vi "Out_Off_N4_201.vi"(4 "Driver Name":T10, 6 "Error Code":T11, 7 "SwitchOFF":T7=TRUE, 8 "error in":T9, 11 "DriverConnect in":T1={"InterfaceType"=enum."VISA", "OpenedSession"="", "InterfaceSettings"={"Interface"=enum."RS232", "EOS 4 read"=enum."LF (\\n)", "EOS 4 write"=enum."LF (\\n)", "TMO, ms"=10000, "Sett"=variant(cluster{"Baud Rate":u32, "Data Bits":u16, "Parity":u16, "Stop Bits":u16, "Flow Control":u16, "Eho":bool} {"Baud Rate"=75, "Data Bits"=0, "Parity"=0, "Stop Bits"=0, "Flow Control"=0, "Eho"=FALSE})}}) -> (0 "error out":T9, 3 "DriverConnect out":T1={"InterfaceType"=enum."VISA", "OpenedSession"="", "InterfaceSettings"={"Interface"=enum."RS232", "EOS 4 read"=enum."LF (\\n)", "EOS 4 write"=enum."LF (\\n)", "TMO, ms"=10000, "Sett"=variant(cluster{"Baud Rate":u32, "Data Bits":u16, "Parity":u16, "Stop Bits":u16, "Flow Control":u16, "Eho":bool} {"Baud Rate"=75, "Data Bits"=0, "Parity"=0, "Stop Bits"=0, "Flow Control"=0, "Eho"=FALSE})}})   [LabVIEW 2018]
uses:
  MOKO_LabViewLibrary/MokoLowLevel/MokoLowLovelControl/MLLC_ErrorCode.ctl
  MOKO_LabViewLibrary/MokoLowLevel/MokoLowLovelControl/MLLC_DriverName.ctl
  MOKO_LabViewLibrary/MokoLowLevel/MokoLowLovelControl/MLLC_Error.ctl
  MOKO_LabViewLibrary/MokoLowLevel/MokoLowLovelControl/MLLC_Delay.ctl
  MOKO_LabViewLibrary/MokoLowLevel/MokoLowLovelControl/MLLC_Boolean.ctl
  MOKO_LabViewLibrary/MokoLowLevel/MokoLowLovelControl/MLLC_Command.ctl
  MOKO_LabViewLibrary/MokoLowLevel/MokoLowLovelControl/MLLC_DriverConnectCluster.ctl
  MOKO_LabViewLibrary/MokoLowLevel/MokoLowLovelControl/MLLC_InterfaceType.ctl
  MOKO_LabViewLibrary/MokoLowLevel/MokoLowLovelControl/MLLC_OpenedSession.ctl
  MOKO_LabViewLibrary/MokoLowLevel/MokoLowLovelControl/MLLC_InterfaceSettings.ctl
  MOKO_LabViewLibrary/MokoLowLevel/MokoLowLovelControl/MLLC_InterfaceKind.ctl
panel:
  out "Array":T6[](array[typedef])
  out "iterations":T8
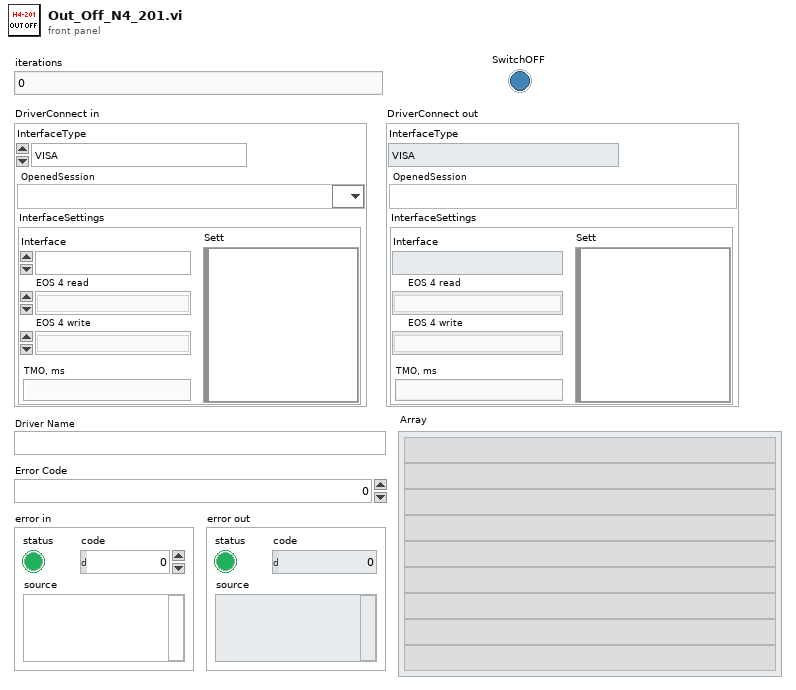
[diagram p1: front panel]
types:
  T1 = typedef "MLLC_DriverConnectCluster.ctl" = cluster{"InterfaceType":T2, "OpenedSession":T3, "InterfaceSettings":T4}
  T2 = typedef "MLLC_InterfaceType.ctl" = enum16{"VISA", "Prologix USB-GPIB"}
  T3 = typedef "MLLC_OpenedSession.ctl" = refnum<visa-resource-name>
  T4 = typedef "MLLC_InterfaceSettings.ctl" = cluster{"Interface":T5, "EOS 4 read":enum16{"Default (=EOS 4 write)", "CR (\\r)", "LF (\\n)", "None"}, "EOS 4 write":enum16{"CR+LF (\\r\\n)", "CR (\\r)", "LF (\\n)", "None"}, "TMO, ms":i32, "Sett":variant}
  T5 = typedef "MLLC_InterfaceKind.ctl" = enum16{"RS232", "GPIB", "USB", "Ethernet", "another"}
  T6 = typedef "MLLC_Command.ctl" = string
  T7 = typedef "MLLC_Boolean.ctl" = bool
  T8 = typedef "MLLC_Delay.ctl" = dbl
  T9 = typedef "MLLC_Error.ctl" = errorcluster
  T10 = typedef "MLLC_DriverName.ctl" = string
  T11 = typedef "MLLC_ErrorCode.ctl" = u32
  T12 = enum16{"Нет симуляции", "В ручную", "Игнорировать"}
  T13 = cluster{"Status":bool, "Error Code":T11, "source":string}
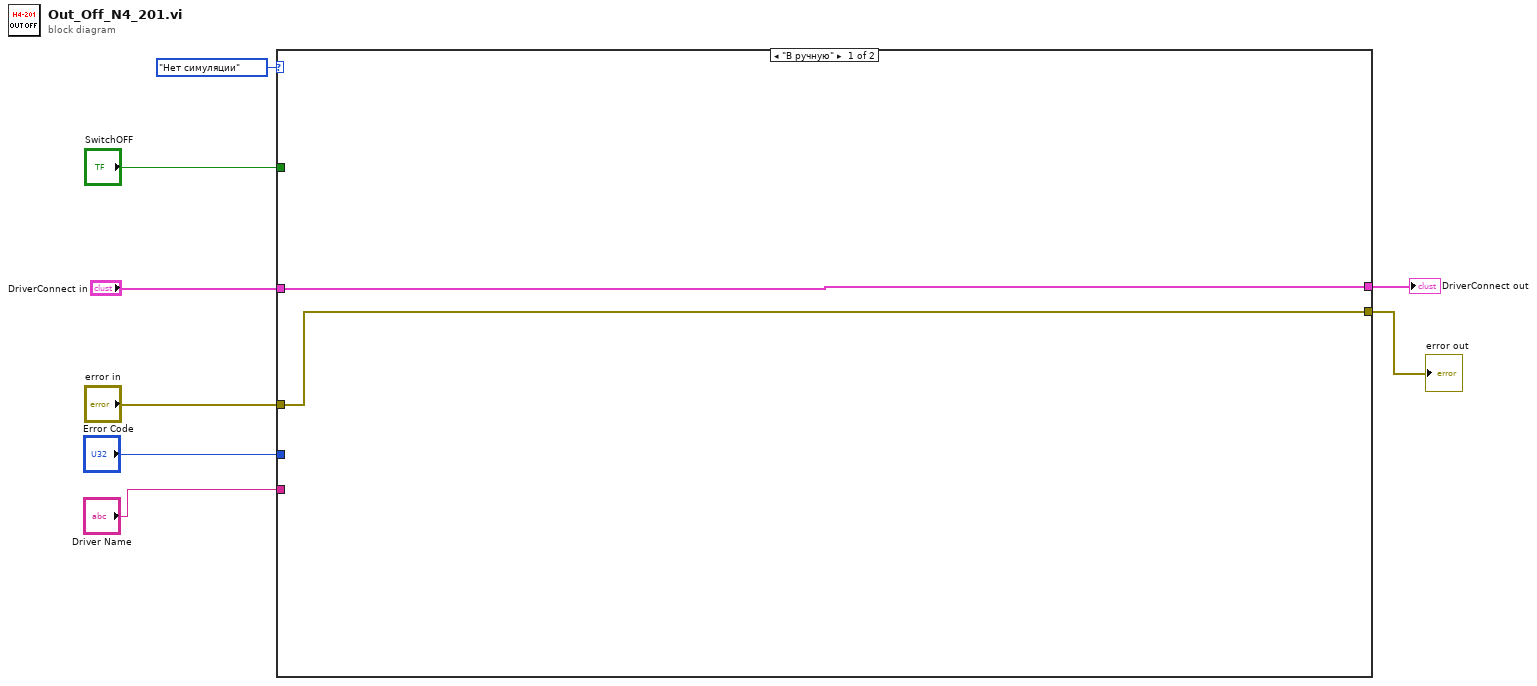
[diagram p0: block diagram]
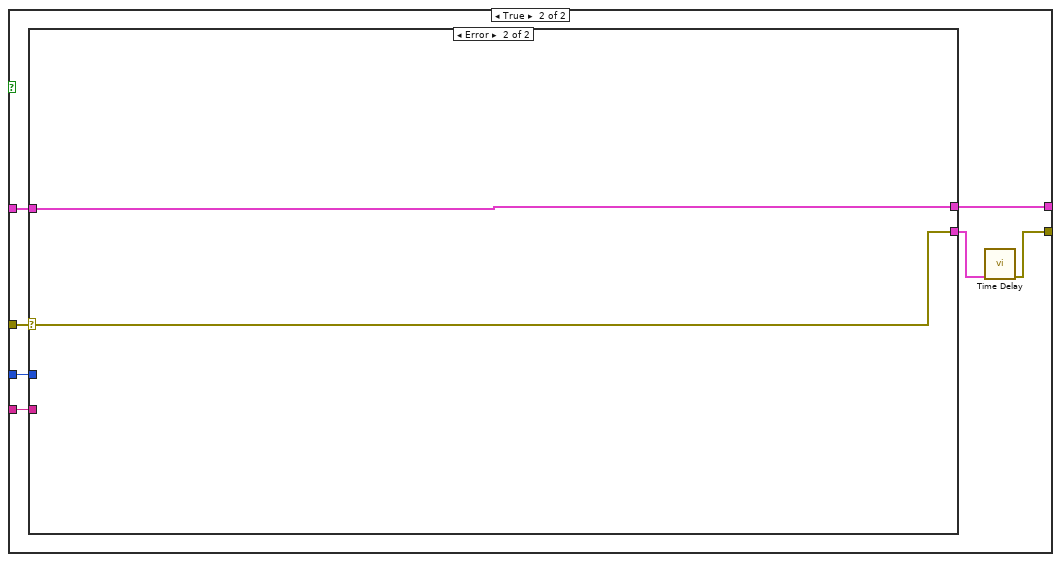
[diagram p3: hidden frame]
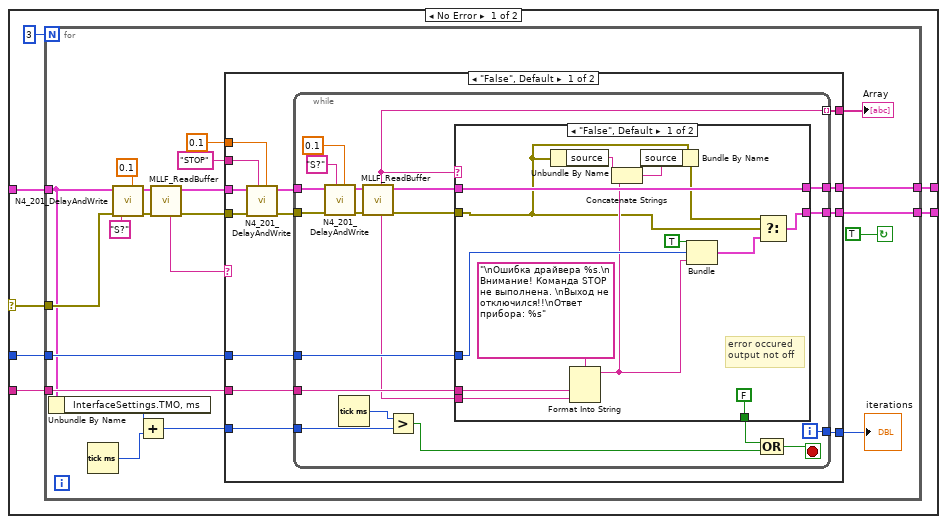
[diagram p4: hidden frame]
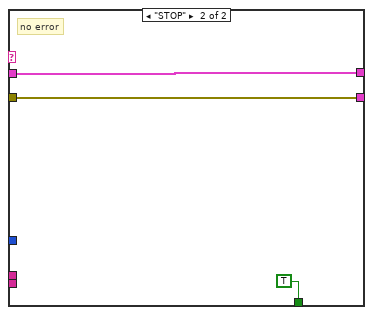
[diagram p5: hidden frame]
diagram:
  n1 = case shown="\"В ручную\"" T12."Нет симуляции" ("Simmulation") {
    tunnel: [w10 w17] -> w1
    tunnel: "Error Code" -> [_ w16]
    tunnel: "Driver Name" -> [_ w15]
    tunnel: "DriverConnect in" -> [w10 w14]
    tunnel: "error in" -> [w9 w13]
    tunnel: "SwitchOFF" -> [_ w12]
    tunnel: [w9 w11] -> w4
    frame "В ручную" {
    }
    frame "Нет симуляции", Default {
      n2 = case shown="False" w12 {
        tunnel: [w18 w20] -> w11
        tunnel: [w19 w26] -> w17
        tunnel: w16 -> [_ w25]
        tunnel: w15 -> [_ w24]
        tunnel: w14 -> [w19 w23]
        tunnel: w13 -> [w18 w22]
        frame False {
        }
        frame True {
          n3 = case shown="Error" w22 {
            selector: w22 -> [w28 w107]
            tunnel: [w33 w107] -> w21
            tunnel: [w32 w106] -> w26
            tunnel: w25 -> [w31 _]
            tunnel: w24 -> [w30 _]
            tunnel: w23 -> [w29 w106]
            frame No Error {
              n4 = for {
                N: 3 -> [_]
                tunnel: [w38] -> w33
                tunnel: [w54] -> w32
                tunnel: w31 -> [w53]
                tunnel: w30 -> [w52]
                tunnel: w29 -> [w34]
                tunnel: w28 -> [w45]
                stop <- TRUE continue-if-true
                n5 = Unbundle By Name(w34) -> ("InterfaceSettings.TMO, ms"=w50:i32)
                n6 = Tick Count (ms)() -> (millisecond timer value=w51:u32)
                n7 = call "N4_201_DelayAndWrite.vi"("Delay Befor (s)"=0.1, "Command"="S?" ("Error Query"), "error in"=w45, "DriverConnect in"=w34) -> ("error out"=w43:T9, "DriverConnect out"=w42:T1)  [unwired: 6 in]
                n8 = Add(x=w50, y=w51) -> (x+y=w49:u32)
                n9 = call "MLLF_ReadBuffer.vi"("Error In"=w43, "DriverConnect in"=w42) -> ("Error Out"=w40:errorcluster, "DriverConnect out"=w41:T1, "String"=w39:string)  [unwired: 6 in]
                n10 = case shown="\"False\", Default" w39 {
                  tunnel: [w67 w105] -> w38
                  tunnel: [w66 w104] -> w54
                  tunnel: w53 -> [w65 _]
                  tunnel: w52 -> [w64 _]
                  tunnel: w49 -> [w63 _]
                  tunnel: [w62 _] -> w48
                  tunnel: [w61 _] -> w36
                  tunnel: "STOP" ("String") -> [w60 _]
                  tunnel: 0.1 ("Delay Befor (s)") -> [w59 _]
                  tunnel: w41 -> [w56 w104]
                  tunnel: w40 -> [w55 w105]
                  frame "False", Default {
                    n11 = call "N4_201_DelayAndWrite.vi"("Delay Befor (s)"=w59, "Command"=w60, "error in"=w55, "DriverConnect in"=w56) -> ("error out"=w57:T9, "DriverConnect out"=w58:T1)  [unwired: 6 in]
                    n12 = while {
                      tunnel: w58 -> [w69]
                      tunnel: w57 -> [w68]
                      tunnel: [w82] -> w67
                      tunnel: [w81] -> w66
                      tunnel: w65 -> [w80]
                      tunnel: w64 -> [w79]
                      tunnel: w63 -> [w77]
                      tunnel: [w73] -> w62
                      tunnel: [w70] -> w61 mode=indexing
                      i -> [w73]
                      stop <- w76 stop-if-true
                      n13 = call "N4_201_DelayAndWrite.vi"("Delay Befor (s)"=0.1, "Command"="S?" ("Error Query"), "error in"=w68, "DriverConnect in"=w69) -> ("error out"=w72:T9, "DriverConnect out"=w86:T1)  [unwired: 6 in]
                      n14 = Tick Count (ms)() -> (millisecond timer value=w78:u32)
                      n15 = call "MLLF_ReadBuffer.vi"("Error In"=w72, "DriverConnect in"=w86) -> ("Error Out"=w83:errorcluster, "DriverConnect out"=w84:T1, "String"=w70:string)  [unwired: 6 in]
                      n16 = Greater?(x=w78, y=w77) -> (0:w74:bool)
                      n17 = case shown="\"False\", Default" w70 {
                        tunnel: w84 -> [w100 w102]
                        tunnel: w83 -> [w91 w103]
                        tunnel: [w88 w103] -> w82
                        tunnel: [w100 w102] -> w81
                        tunnel: w80 -> [w97 _]
                        tunnel: w79 -> [w96 _]
                        tunnel: [FALSE TRUE] -> w75
                        tunnel: w70 -> [w89 _]
                        frame "False", Default {
                          # "error occured\noutput not off"
                          n18 = Unbundle By Name(w91) -> ("source"=w93:string)
                          n19 = Format Into String(format string="\nОшибка драйвера %s.\n Внимание! Команда STOP не выполнена. \nВыход не отключился!!\nОтвет прибора: %s", w96, w89) -> (resulting string=w92:string)  [unwired: 2 in, 1 out]
                          n20 = Concatenate Strings(w93, w92) -> (w94:string)
                          n21 = Bundle By Name(cluster=w91, "source"=w94) -> (w90:errorcluster)
                          n22 = Bundle("Status"=TRUE, "Error Code"=w97, w92) -> (w87:cluster{"Status":bool, "Error Code":T11, string})  [unwired: 1 in]
                          n23 = Select(t=w90, s=w91, f=w87) -> (s? t:f=w88:T13)
                        }
                        frame "STOP" {
                          # "no error"
                        }
                      }
                      n24 = Compound Arithmetic op=OR(w75, w74) -> (w76:bool)
                    }
                  }
                  frame "stop" {
                  }
                }
                "iterations" <- w48
                "Array" <- w36
              }
            }
            frame Error {
            }
          }
          n25 = call "Time Delay"("error in (no error)"=w21) -> ("error out"=w20:errorcluster)  [unwired: 10 in]
        }
      }
    }
  }
  "error out" <- w4
  "DriverConnect out" <- w1
